vi "Vision Server Remove Vision Update.vi"(0 "Vision Server":T1={"connection ID"=refnum, "Running?"=TRUE, "TCP Port"=65535, "LastMessageReceivedTime"=0.0, "WantsAppRestart"=FALSE, "IsConnect"=FALSE, "Targets Updates"=[{"Valid?"=FALSE, "CapturedAtTimestamp"=0.0, "Targets Message"={"capturedAgoMs"=0, "targets"=[{"x"=0.0, "y"=0.0, "z"=0.0, "theta"=0.0}]}}]}, 1 "Targets Update":T2={"Valid?"=FALSE, "CapturedAtTimestamp"=0.0, "Targets Message"={"capturedAgoMs"=0, "targets"=[{"x"=0.0, "y"=0.0, "z"=0.0, "theta"=0.0}]}}) -> (2 "Vision Server":T1={"connection ID"=refnum, "Running?"=TRUE, "TCP Port"=65535, "LastMessageReceivedTime"=0.0, "WantsAppRestart"=FALSE, "IsConnect"=FALSE, "Targets Updates"=[{"Valid?"=FALSE, "CapturedAtTimestamp"=0.0, "Targets Message"={"capturedAgoMs"=0, "targets"=[{"x"=0.0, "y"=0.0, "z"=0.0, "theta"=0.0}]}}]})   [LabVIEW 2016]
uses:
  Vision Server.ctl
  Messages/Targets/Targets Update.ctl
  Messages/Targets/Targets Message.ctl
  Messages/Targets/Targets Info.ctl
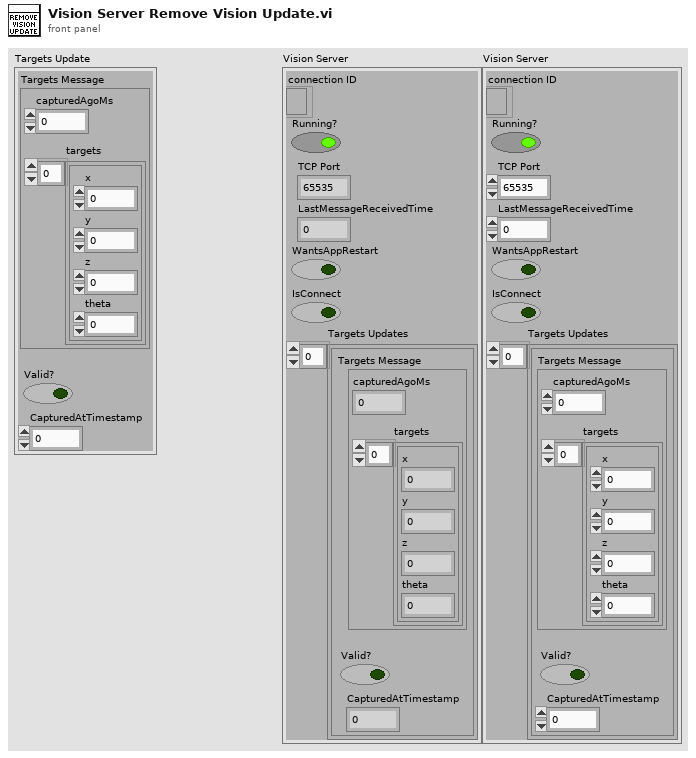
[diagram p1: front panel]
types:
  T1 = typedef "Vision Server.ctl" = cluster{"connection ID":refnum<k5>, "Running?":bool, "TCP Port":u16, "LastMessageReceivedTime":dbl, "WantsAppRestart":bool, "IsConnect":bool, "Targets Updates":T2[]}
  T2 = typedef "Targets Update.ctl" = cluster{"Valid?":bool, "CapturedAtTimestamp":dbl, "Targets Message":T3}
  T3 = typedef "Targets Message.ctl" = cluster{"capturedAgoMs":i32, "targets":T4[]}
  T4 = typedef "Targets Info.ctl" = cluster{"x":dbl, "y":dbl, "z":dbl, "theta":dbl}
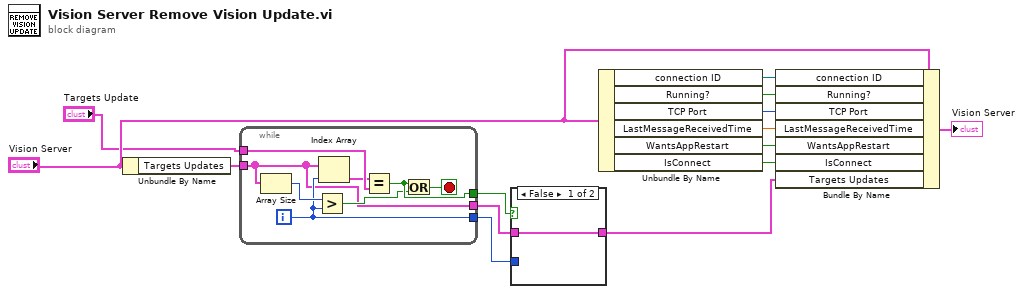
[diagram p0: block diagram]
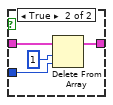
[diagram p2: hidden frame]
diagram:
  n1 = Unbundle By Name("Vision Server") -> ("Targets Updates"=w14:T2[])
  n2 = while {
    tunnel: w14 -> [w15]
    tunnel: "Targets Update" -> [w22]
    tunnel: [w16] -> w11
    tunnel: [w20] -> w13
    tunnel: [w15] -> w12
    i -> [w16]
    stop <- w19 stop-if-true
    n3 = Array Size(array=w15) -> (size(s)=w17:i32)
    n4 = Greater?(x=w17, y=w16) -> (0:w18:bool)
    n5 = Index Array(array=w15, index=w16) -> (element=w21:T2)
    n6 = Equal?(x=w21, y=w22) -> (x = y?=w20:bool)
    n7 = Or(x=w20, y=w18) -> (x .or. y?=w19:bool)
  }
  n8 = case shown="False" w13 {
    tunnel: w12 -> [w23 w27]
    tunnel: w11 -> [_ w25]
    tunnel: [w23 w24] -> w4
    frame False {
    }
    frame True {
      n9 = Delete From Array(array=w27, length=1, index=w25) -> (array with subset deleted=w24:T2[])  [unwired: 1 out]
    }
  }
  n10 = Unbundle By Name("Vision Server") -> ("connection ID"=w10:refnum<k5>, "Running?"=w9:bool, "TCP Port"=w8:u16, "LastMessageReceivedTime"=w7:dbl, "WantsAppRestart"=w6:bool, "IsConnect"=w5:bool)
  n11 = Bundle By Name(cluster="Vision Server", "connection ID"=w10, "Running?"=w9, "TCP Port"=w8, "LastMessageReceivedTime"=w7, "WantsAppRestart"=w6, "IsConnect"=w5, "Targets Updates"=w4) -> (→"Vision Server":T1)
